vi "Instr_InitObject.vi"(8 "error in (no error)":errorcluster, 9 "Instrument Configuration":variant, 10 "GPIB address":string, 11 "KE2657A in":refnum<class "KE2657A.lvclass">) -> (0 "error out":errorcluster, 3 "KE2657A out":refnum<class "KE2657A.lvclass">)   [LabVIEW 2018, in "KE2657A.lvclass"]
uses:
  KE2657A.lvclass
  InstrumentSetup.vi
  KE2657A_CommandsGlobal.vi
  SupplyControl.lvclass
  InstrControl.lvclass
  <instrlib>/Keithley 2600 Series/Keithley 2600 Series.lvlib
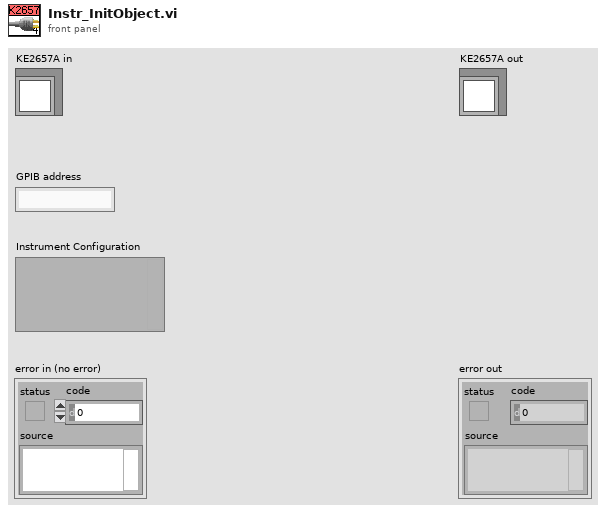
[diagram p1: front panel]
types:
  T1 = cluster{"Current Limit":sgl, "Compliance":u16, "Range:":u16, "KE2657A":refnum<class "KE2657A.lvclass">}
  T2 = cluster{"Instrument name":string, "Command \"Reset\"":string, "Command \"Initialise\"":string, "Command \"Arm\"":string, "Command \"SetVolts\"":string, "Command \"Compliance?\"":string, "Command \"Standby\"":string, "Command \"Read Current\"":string}
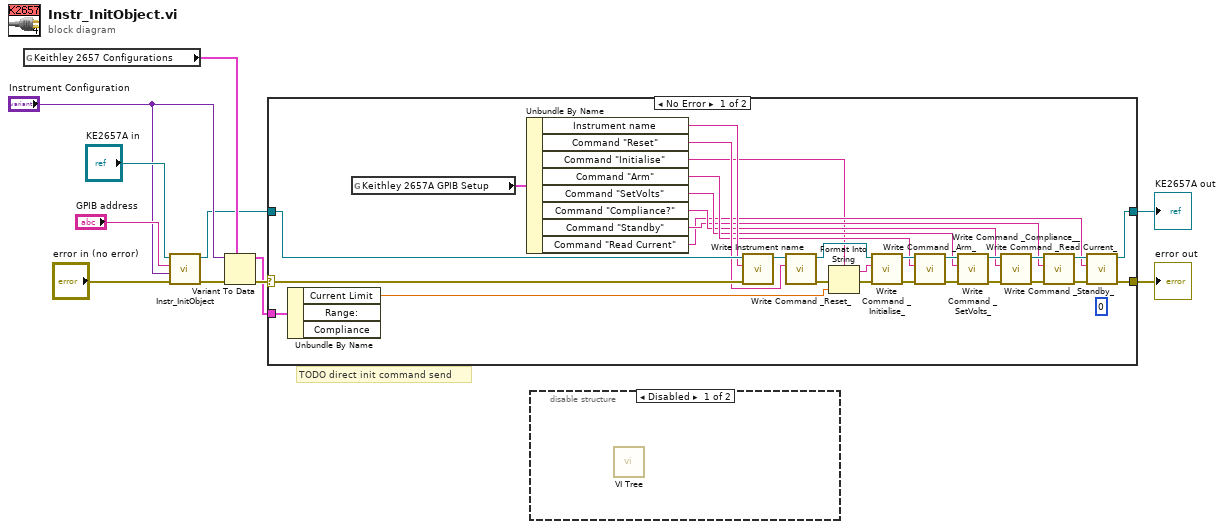
[diagram p0: block diagram]
diagram:
  # "TODO direct init command send"
  n1 = global read "InstrumentSetup.vi" "Keithley 2657 Configurations"() -> (w8:T1)
  n2 = call-parent "Instr_InitObject.vi"("error in (no error)"="error in (no error)", "Instrument Configuration"="Instrument Configuration", "GPIB address"="GPIB address", "SupplyControl in"="KE2657A in") -> ("error out"=w6:errorcluster, "SupplyControl out"=w3:refnum<class "KE2657A.lvclass">)  [unwired: 6 in]
  n3 = Variant To Data(error in=w6, type=w8, Variant="Instrument Configuration") -> (data=w4:T1, error out=w5:errorcluster)
  n4 = case shown="No Error" w5 {
    selector: w5 -> [w37 w42]
    tunnel: w4 -> [w41 _]
    tunnel: w3 -> [w39 w43]
    tunnel: [w18 w43] -> w2
    tunnel: [w17 w42] -> w1
    frame No Error {
      (unwired) u16 0 ("Range:")
      n5 = Unbundle By Name(w41) -> ("Current Limit"=w13:sgl)  [unwired: 2 out]
      n6 = global read "KE2657A_CommandsGlobal.vi" "Keithley 2657A GPIB Setup"() -> (w40:T2)
      n7 = Unbundle By Name(w40) -> ("Instrument name"=w38:string, "Command \"Reset\""=w24:string, "Command \"Initialise\""=w16:string, "Command \"Arm\""=w23:string, "Command \"SetVolts\""=w22:string, "Command \"Compliance?\""=w21:string, "Command \"Standby\""=w20:string, "Command \"Read Current\""=w19:string)
      n8 = call-dynamic "Write Instrument name.vi"("error in (no error)"=w37, "Instrument name"=w38, "InstControl in"=w39) -> ("InstControl out"=w25:refnum<class "KE2657A.lvclass">)  [unwired: 7 in, 1 out]
      n9 = call-dynamic "Write Command _Reset_.vi"("Command \"Reset\""=w24, "SupplyControl in"=w25) -> ("error out"=w14:errorcluster, "SupplyControl out"=w36:refnum<class "KE2657A.lvclass">)  [unwired: 8 in]
      n10 = Format Into String(format string=w16, error in=w14, w13) -> (resulting string=w12:string, error out=w15:errorcluster)  [unwired: 1 in]
      n11 = call-dynamic "Write Command _Initialise_.vi"("error in (no error)"=w15, "Command \"Initialise\""=w12, "SupplyControl in"=w36) -> ("error out"=w30:errorcluster, "SupplyControl out"=w35:refnum<class "KE2657A.lvclass">)  [unwired: 7 in]
      n12 = call-dynamic "Write Command _Arm_.vi"("error in (no error)"=w30, "Command \"Arm\""=w23, "SupplyControl in"=w35) -> ("error out"=w29:errorcluster, "SupplyControl out"=w34:refnum<class "KE2657A.lvclass">)  [unwired: 7 in]
      n13 = call-dynamic "Write Command _SetVolts_.vi"("error in (no error)"=w29, "Command \"SetVolts\""=w22, "SupplyControl in"=w34) -> ("error out"=w28:errorcluster, "SupplyControl out"=w33:refnum<class "KE2657A.lvclass">)  [unwired: 7 in]
      n14 = call-dynamic "Write Command _Compliance__.vi"("error in (no error)"=w28, "Command \"Compliance?\""=w21, "SupplyControl in"=w33) -> ("error out"=w27:errorcluster, "SupplyControl out"=w32:refnum<class "KE2657A.lvclass">)  [unwired: 7 in]
      n15 = call-dynamic "Write Command _Standby_.vi"("error in (no error)"=w27, "Command \"Standby\""=w20, "SupplyControl in"=w32) -> ("error out"=w26:errorcluster, "SupplyControl out"=w31:refnum<class "KE2657A.lvclass">)  [unwired: 7 in]
      n16 = call-dynamic "Write Command _Read Current_.vi"("error in (no error)"=w26, "Command \"Read Current\""=w19, "SupplyControl in"=w31) -> ("error out"=w17:errorcluster, "SupplyControl out"=w18:refnum<class "KE2657A.lvclass">)  [unwired: 7 in]
    }
    frame Error {
    }
  }
  "error out" <- w1
  "KE2657A out" <- w2
  n17 = disable-structure shown="Disabled" {
    frame Disabled {
      n18 = call <instrlib>:"VI Tree.vi"() -> ()  [unwired: 12 in]
    }
    frame Enabled {
    }
  }
